vi "Initialise List Box.vi"(11 "Main Display in":refnum<class "Main Display.lvclass">) -> (0 "error out":errorcluster)   [LabVIEW 2016, in "Assert API Components.lvlib" / "Assert Display.lvlib" / "Main Display.lvlib" / "Main Display.lvclass"]
uses:
  Main Display.lvclass
  C:/Program Files (x86)/National Instruments/LabVIEW 2016/vi.lib/ActorFramework/Actor/Actor.lvclass
  Actions.ctl
  <vilib>/ActorFramework/Actor/Actor.lvclass/Actor.ctl
  <vilib>/ActorFramework/Message Enqueuer/Message Enqueuer.lvclass/Message Enqueuer.ctl
  Main Display.lvclass/Main Display.ctl
  Display Configurations/Base Display Configuration.lvclass/Base Display Configuration.ctl
  Main Display Messages/Do Action Msg/Do Action Msg.lvclass/Do Action Msg.ctl
  <vilib>/ActorFramework/Message Enqueuer/Init from Existing Queue.vi
  <vilib>/ActorFramework/Message Enqueuer/Enqueue.vi
  Main Display Messages/Do Action Msg/Do Action Msg.lvclass
  C:/Program Files (x86)/National Instruments/LabVIEW 2016/vi.lib/ActorFramework/Message/Message.lvclass
  <vilib>/Utility/LVClass/Get LV Class Name.vi
  <resource>/AFDebug/Generate Trace for Message.vi
  <vilib>/ActorFramework/Message Priority Queue/Priority Enqueue.vi
  <vilib>/ActorFramework/Message Enqueuer/Message Enqueuer.lvclass
  <vilib>/ActorFramework/Actor/Actor.lvclass
  Display Configurations/Base Display Configuration.lvclass
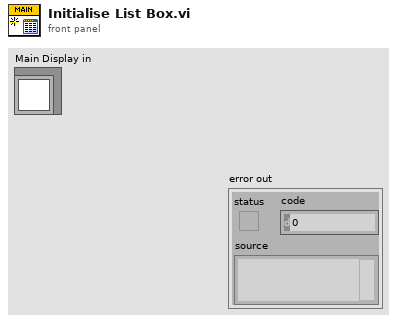
[diagram p1: front panel]
types:
  T1 = typedef "Assert API Components.lvlib/Assert Display.lvlib/Main Display.lvlib/Main Display.lvclass/Actions.ctl" = enum16{"Update Column Headers", "Update Timeout"}
  T2 = typedef "Assert API Components.lvlib/Assert Display.lvlib/Main Display.lvlib/Display Colours.ctl" = cluster{"Enable Colours":bool, "Passed Colour":u32, "Failed Colour":u32}
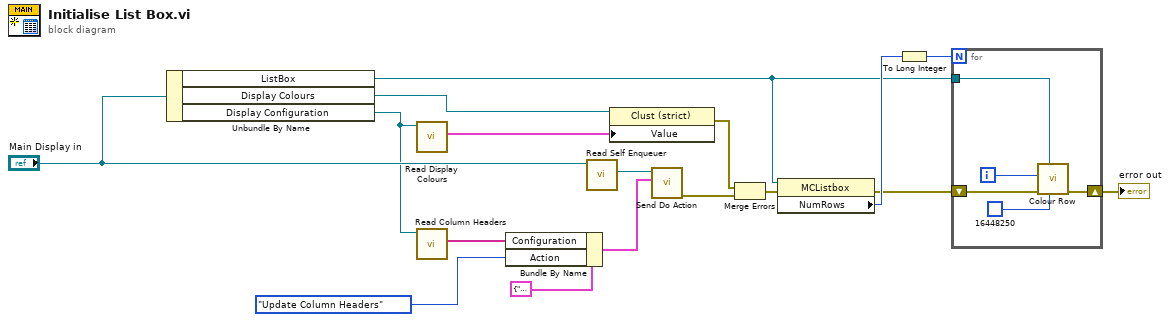
[diagram p0: block diagram]
diagram:
  n1 = Unbundle By Name("Main Display in") -> ("ListBox"=w1:refnum<vi>, "Display Colours"=w4:refnum<vi>, "Display Configuration"=w7:refnum<class "Base Display Configuration.lvclass">)
  n2 = call "Read Display Colours.vi"("Base Display Configuration in"=w7) -> ("Display Colours"=w3:T2)  [unwired: 10 in]
  n3 = call "Read Column Headers.vi"("Base Display Configuration in"=w7) -> ("Column Headers"=w14:string[])  [unwired: 10 in]
  n4 = Bundle By Name(cluster=cluster{"Action":T1, "Configuration":variant} {"Action"=enum."Update Column Headers", "Configuration"=variant} ("Action Configuration"), "Configuration"=w14, "Action"=Actions."Update Column Headers") -> (w15:cluster{"Action":T1, "Configuration":variant})
  n5 = call <vilib>:"Read Self Enqueuer.vi"("Actor"="Main Display in") -> ("Self Enqueuer"=w5:refnum<class "Message Enqueuer.lvclass">)  [unwired: 10 in]
  n6 = property class="Clust (strict)"(reference=w4, "Value"=w3) -> (error out=w2:errorcluster)  [unwired: 1 in, 1 out]
  n7 = call "Send Do Action.vi"("Action Configuration"=w15, "Message Enqueuer"=w5) -> ("error out"=w10:errorcluster)  [unwired: 8 in, 1 out]
  n8 = Merge Errors(w2, w10) -> (w6:errorcluster)
  n9 = property class="MCListbox"(reference=w1, error in=w6) -> (error out=w11:errorcluster, "NumRows"=w12:u32)  [unwired: 1 out]
  n10 = To Long Integer(number=w12) -> (32bit integer=w13:i32)
  n11 = for {
    N: w13 -> [_]
    tunnel: w1 -> [w18]
    shift-right: [w21] -> w9
    shift-left: w11 -> [w22]
    i -> [w20]
    n12 = call "Colour Row.vi"("Row Colour"=u32 16448250, "MulticolumnListbox in"=w18, "error in (no error)"=w22, "Row Number"=w20) -> ("error out"=w21:errorcluster)  [unwired: 7 in]
  }
  "error out" <- w9
